vi "Write Key.vi"(2 "Data":string[](array[string]), 3 "Key name":string[](array[string]), 4 "section":string caption="段") -> (0 "查询结果":bool[](array[boolean]), 1 "查询":T1)   [LabVIEW 2014]
uses:
  <vilib>/Utility/config.llb/Write Key (String).vi
  <vilib>/Utility/config.llb/NI_LVConfig.lvlib
panel:
  out "未知健":bool
  out "error out":errorcluster caption="错误输出"
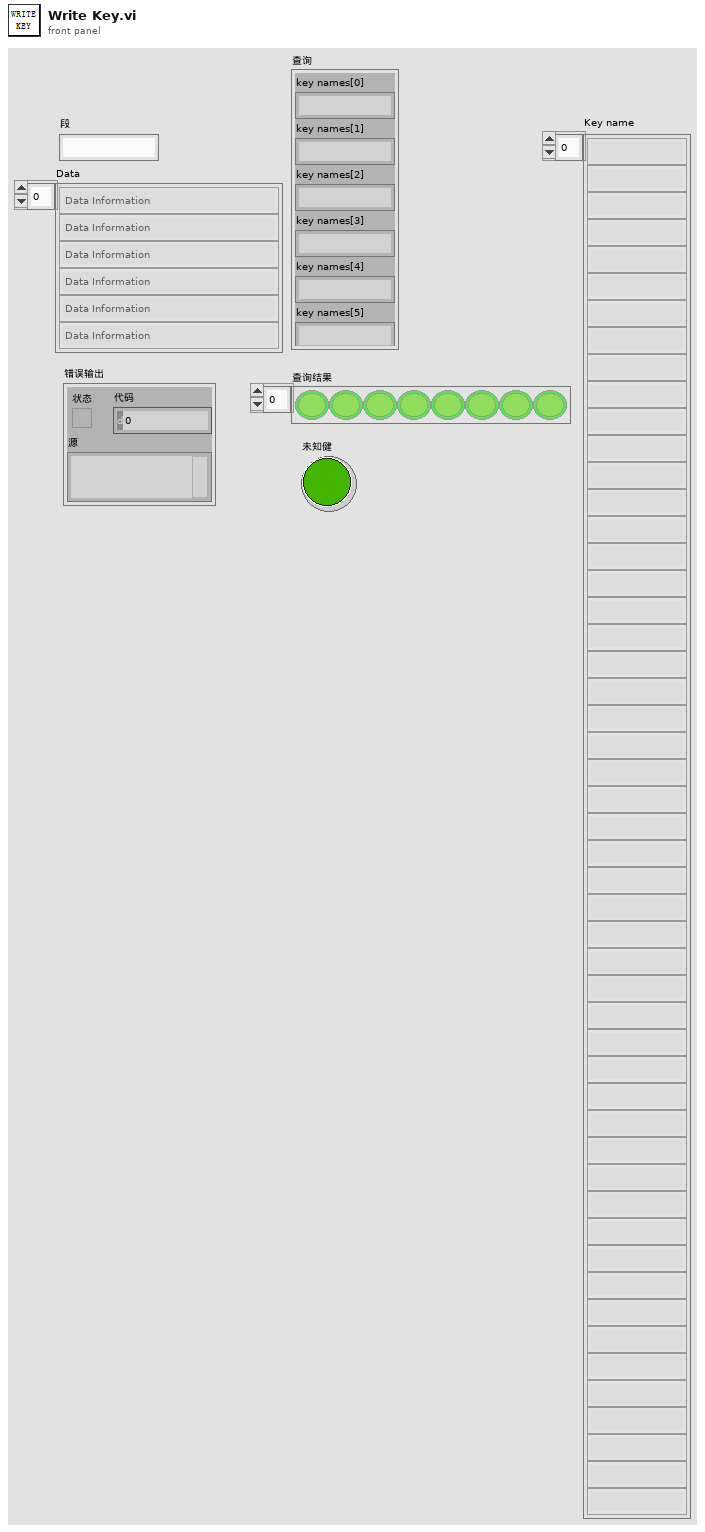
[diagram p1: front panel]
types:
  T1 = cluster{"key names[0]":string, "key names[1]":string, "key names[2]":string, "key names[3]":string, "key names[4]":string, "key names[5]":string, "key names[6]":string, "key names[7]":string, "key names[8]":string}
  T2 = typedef "NI_LVConfig.lvlib/Config Data RefNum.ctl" = refnum<k1>
  T3 = cluster{"[0]":bool, "[1]":bool, "[2]":bool, "[3]":bool, "[4]":bool, "[5]":bool, "[6]":bool, "[7]":bool, "[8]":bool}
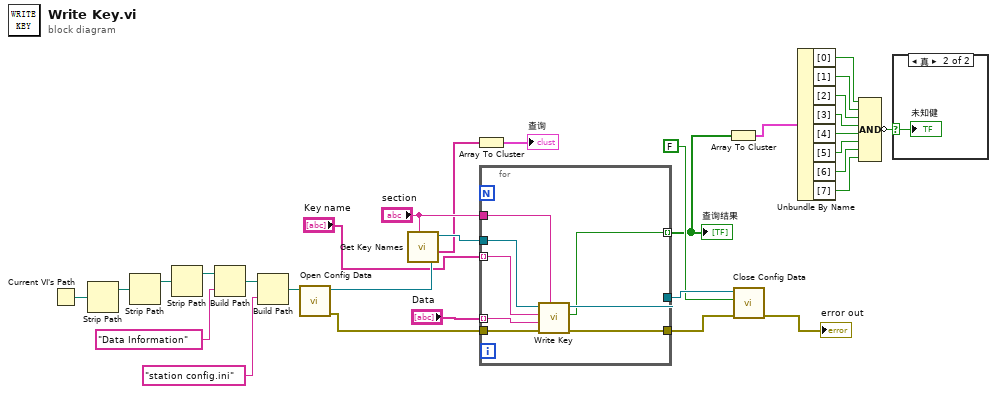
[diagram p0: block diagram]
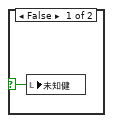
[diagram p2: hidden frame]
diagram:
  n1 = Current VI's Path() -> (path=w25:path)
  n2 = Strip Path(path=w25) -> (stripped path=w26:path)  [unwired: 1 out]
  n3 = Strip Path(path=w26) -> (stripped path=w30:path)  [unwired: 1 out]
  n4 = Strip Path(path=w30) -> (stripped path=w31:path)  [unwired: 1 out]
  n5 = Build Path(base path=w31, name or relative path="Data Information" ("名称或相对路径")) -> (appended path=w28:path)
  n6 = Build Path(base path=w28, name or relative path="station config.ini" ("名称或相对路径")) -> (appended path=w24:path)
  n7 = call <vilib>:"Open Config Data.vi"("configuration file path"=w24) -> ("error out"=w23:errorcluster, "refnum"=w17:T2)  [unwired: 8 in, 1 out]
  n8 = call <vilib>:"Get Key Names.vi"("section"="section", "refnum"=w17) -> ("key names"=w15:string[], "refnum out"=w16:T2)  [unwired: 6 in, 2 out]
  n9 = Array To Cluster(array=w15) -> (cluster=→"查询":T1)
  n10 = for {
    tunnel: "section" -> [w36]
    tunnel: w23 -> [w39]
    tunnel: [w37] -> w20
    tunnel: w16 -> [w35]
    tunnel: [w38] -> w22
    tunnel: "Key name" -> [w34] mode=indexing
    tunnel: "Data" -> [w33] mode=indexing
    tunnel: [w32] -> w2 mode=indexing
    n11 = call-poly <vilib>:"Write Key.vi"("section"=w36, "error in (no error)"=w39, "value"=w33, "key"=w34, "refnum"=w35) -> ("error out"=w37:errorcluster, "found?"=w32:bool, "refnum out"=w38:T2)  [unwired: 4 in]
  }
  "查询结果" <- w2
  n12 = Array To Cluster(array=w2) -> (cluster=w3:T3)
  n13 = call <vilib>:"Close Config Data.vi"("error in (no error)"=w20, "write file if changed (T)"=FALSE, "refnum"=w22) -> ("error out"=→"error out":errorcluster)  [unwired: 7 in, 1 out]
  n14 = Unbundle By Name(w3) -> ("[0]"=w12:bool, "[1]"=w11:bool, "[2]"=w10:bool, "[3]"=w9:bool, "[4]"=w8:bool, "[5]"=w7:bool, "[6]"=w6:bool, "[7]"=w5:bool)
  n15 = Compound Arithmetic op=AND(w12, w11, w10, w9, w8, w7, w6, w5) -> (invert w4:bool)
  n16 = case shown="真" w4 {
    selector: w4 -> [w40 w41]
    frame False {
      n17 = local write "未知健"(w40) -> ()
    }
    frame True {
      "未知健" <- w41
    }
  }
